vi "Danger Array_Update.vi"(8 "Value":i32, 9 "Column":i32, 10 "Row":i32, 11 "AntFarm_MB":refnum<class "AntFarm_MB.lvclass">) -> (3 "AntFarm_MB Out":refnum<class "AntFarm_MB.lvclass">)   [LabVIEW 2017, in "AntFarm_MB.lvclass"]
uses:
  AntFarm_MB.lvclass
  AntFarm_MB.lvclass/AntFarm_MB.ctl
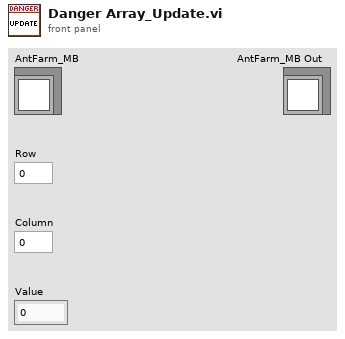
[diagram p1: front panel]
types:
  T1 = typedef "Cluster_Ant Farm Global Data.ctl" = cluster{"Move Map":i32[][], "Danger Map":i32[][], "Attack Rows":i32[], "Attack Columns":i32[], "Square count":i32, "Last Round":i32, "Danger Threshold":i32}
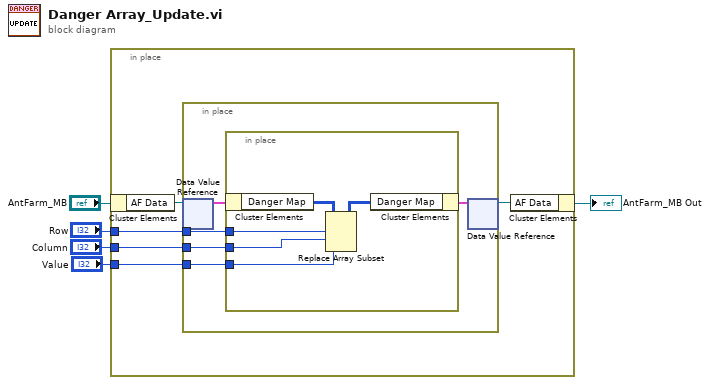
[diagram p0: block diagram]
diagram:
  n1 = in-place {
    in-place-border: "Row" -> [w8]
    in-place-border: "Column" -> [w7]
    in-place-border: "Value" -> [w6]
    n2 = in-place-cluster #1("AntFarm_MB") -> ("AF Data"=w10:refnum<data-value>)
    n3 = in-place {
      in-place-border: w8 -> [w15]
      in-place-border: w7 -> [w14]
      in-place-border: w6 -> [w13]
      n4 = in-place-dvr #2(w10) -> (w12:T1)  [unwired: 1 out]
      n5 = in-place {
        in-place-border: w15 -> [w20]
        in-place-border: w14 -> [w19]
        in-place-border: w13 -> [w18]
        n6 = in-place-cluster #3(w12) -> ("Danger Map"=w17:i32[][])
        n7 = Replace Array Subset(array=w17, new element=w18, index (row)=w20, index (col)=w19) -> (w16:i32[][])
        n8 = in-place-cluster #3("Danger Map"=w16) -> (w11:T1)
      }
      n9 = in-place-dvr #2(w11) -> (w9:refnum<data-value>)  [unwired: 1 out]
    }
    n10 = in-place-cluster #1("AF Data"=w9) -> (→"AntFarm_MB Out":refnum<class "AntFarm_MB.lvclass">)
  }
